vi "全局 时间2.vi"() -> ()   [LabVIEW 2016]
panel:
  in  "时间2":string
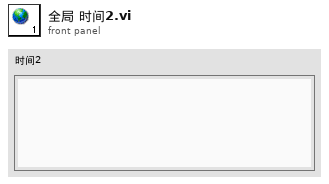
[diagram p1: front panel]
diagram:
